vi "compare typedefs.vi"() -> ()   [LabVIEW 2017]
uses:
  Type Defs/ECAT Channel Data Type.ctl
  Scan Engine Custom Device.lvlib
  Type Defs/UDV Data Type.ctl
panel:
  in  "UDV Data Type 2":T1
  in  "UDV Data Type":T2=enum."SGL"
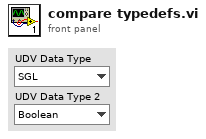
[diagram p1: front panel]
types:
  T1 = typedef "Scan Engine Custom Device.lvlib/UDV Data Type.ctl" = enum16{"Boolean", "Fixed Point", "Int8", "Int16", "Int32", "Int64", "U32 Bit Field", "UInt8", "UInt16", "UInt32", "UInt64", "Other"}
  T2 = typedef "Scan Engine Custom Device.lvlib/ECAT Channel Data Type.ctl" = enum16{"Boolean", "Fixed Point", "Int8", "Int16", "Int32", "Int64", "U32 Bit Field", "UInt8", "UInt16", "UInt32", "UInt64", "Other", "DBL", "SGL"}
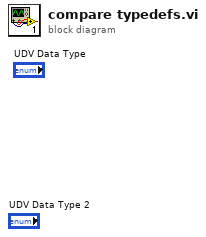
[diagram p0: block diagram]
diagram:
